vi "Create Object.vi"(9 "Self Msg Q":refnum<class "Msg Q.lvclass">, 10 "Call Msg Q":refnum<class "Msg Q.lvclass">) -> (3 "Self Actor out":refnum<class "Self Actor.lvclass">)   [LabVIEW 2021, in "LVCAM.lvlib" / "Self Actor.lvclass"]
uses:
  Self Actor.lvclass
  Msg Q/Msg Q.lvclass
  Self Actor.lvclass/Self Actor.ctl
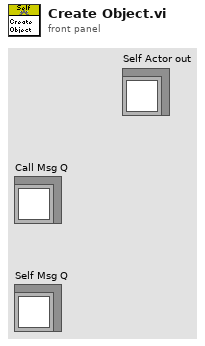
[diagram p1: front panel]
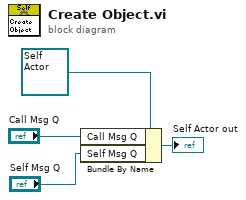
[diagram p0: block diagram]
diagram:
  n1 = Bundle By Name(cluster=refnum<class "Self Actor.lvclass"> refnum ("Self Actor in"), "Call Msg Q"="Call Msg Q", "Self Msg Q"="Self Msg Q") -> (→"Self Actor out":refnum<class "Self Actor.lvclass">)
